vi "ChanotchPassBand.vi"(5 "Half band width":dbl, 8 "Continuum":enum16{"Keep Continuum", "Remove Continuum"}(ring), 9 "Sample/fringe":dbl, 13 "Signal":dbl[](array[numeric])) -> (2 "Chanotched Signal":dbl[](array[numeric]))   [LabVIEW 2009]
uses:
  <vilib>/Analysis/NI_AALBase.lvlib
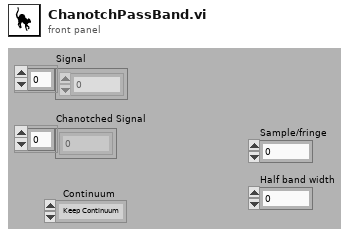
[diagram p1: front panel]
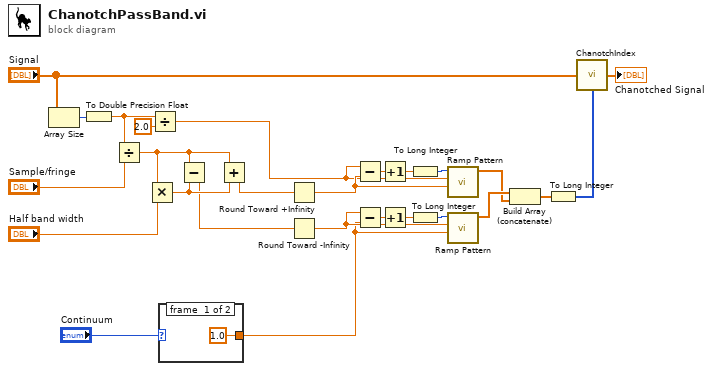
[diagram p0: block diagram]
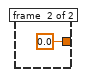
[diagram p2: hidden frame]
diagram:
  n1 = Array Size(array="Signal") -> (size(s)=w24:i32)
  n2 = To Double Precision Float(number=w24) -> (double precision float=w9:dbl)
  n3 = Divide(x=w9, y="Sample/fringe") -> (x/y=w21:dbl)
  n4 = Multiply(x=w21, y="Half band width") -> (x*y=w20:dbl)
  n5 = Divide(x=w9, y=2.0) -> (x/y=w7:dbl)
  n6 = case shown="\"Keep Continuum\"" "Continuum" {
    tunnel: [1.0 ("start") 0.0 ("start")] -> w1
    frame #0 {
    }
    frame #1 {
    }
  }
  n7 = Subtract(x=w21, y=w20) -> (x-y=w19:dbl)
  n8 = Add(x=w21, y=w20) -> (x+y=w11:dbl)
  n9 = Round Toward +Infinity(x=w11) -> (ceil(x): smallest int >= x=w10:dbl)
  n10 = Round Toward -Infinity(1:w19) -> (0:w15:dbl)
  n11 = Subtract(x=w7, y=w10) -> (x-y=w14:dbl)
  n12 = Subtract(x=w15, y=w1) -> (x-y=w16:dbl)
  n13 = Increment(x=w14) -> (x+1=w12:dbl)
  n14 = Increment(x=w16) -> (x+1=w18:dbl)
  n15 = To Long Integer(number=w12) -> (32bit integer=w13:i32)
  n16 = To Long Integer(number=w18) -> (32bit integer=w17:i32)
  n17 = call <vilib>:"Ramp Pattern.vi"("start"=w10, "end"=w7, "samples"=w13) -> ("Ramp Pattern"=w3:dbl[])  [unwired: 7 in, 1 out]
  n18 = call <vilib>:"Ramp Pattern.vi"("start"=w1, "end"=w15, "samples"=w17) -> ("Ramp Pattern"=w4:dbl[])  [unwired: 7 in, 1 out]
  n19 = Build Array (concatenate)(w4, w3) -> (w6:dbl[])
  n20 = To Long Integer(number=w6) -> (32bit integer=w5:i32[])
  n21 = call "ChanotchIndex.vi"("Signal"="Signal", "Freq"=w5) -> ("Chanotched Signal"=→"Chanotched Signal":dbl[])
